vi "wait on clock.vi"(8 "error in":errorcluster, 10 "dt":u32=1, 11 "timing source in":refnum<class "DAQmx Single Point HW Timed.lvclass">) -> (0 "error out":errorcluster, 2 "ticks since last call":u32, 3 "timing source out":refnum<class "DAQmx Single Point HW Timed.lvclass">)   [LabVIEW 2014, in "DAQmx Single Point HW Timed.lvclass"]
doc: "This core timing function is used inside of a loop to wait for a clock signal, or dt ticks of a clock signal."
uses:
  DAQmx Single Point HW Timed.lvclass
  <vilib>/NI/Module Timing Source/timing source/TBM timing source.lvclass
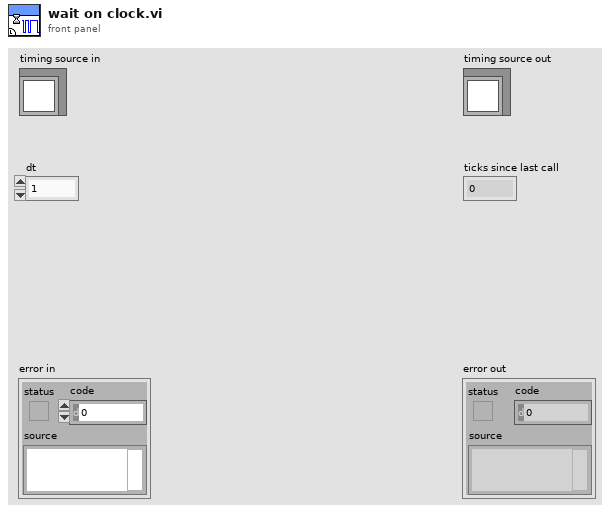
[diagram p1: front panel]
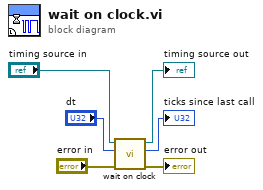
[diagram p0: block diagram]
diagram:
  n1 = call-parent "wait on clock.vi"("error in"="error in", "dt"="dt", "timing source in"="timing source in") -> ("error out"=→"error out":errorcluster, "ticks since last call"=→"ticks since last call":u32, "timing source out"=→"timing source out":refnum<class "DAQmx Single Point HW Timed.lvclass">)  [unwired: 6 in]
